vi "Stop Core.vi"(10 "final error code":i32, 11 "Valve in":refnum<class "Valve.lvclass">) -> (3 "Valve out":refnum<class "Valve.lvclass">)   [LabVIEW 2015, in "cRIO-Carbondioxide.lvlib" / "CO2-Actor.lvlib" / "Valve.lvclass"]
doc: "(<B>Filename</B>: Actor Framework.lvlib:Actor.lvclass:Stop Core.vi)\n\nDefines what the actor does before it stops. Use the <B>final error code</B> input to determine whether the actor shut down in response to an error.\n\nBy default, this method does nothing. A descendant class may override it to define behavior, such as shutting down any processes the actor initiated in its override of the Actor Core method."
uses:
  Valve.lvclass
  Valve.lvclass/Valve.ctl
  Interlocks/Interlock Bool/Interlock Bool.lvclass
  CO2 Actor/CO2 Actor.lvclass/CO2 Actor.ctl
  Interlocks/Interlock Chain/Interlock Chain.lvclass/Interlock Chain.ctl
  Interlocks/Interlock/Interlock.lvclass/Interlock.ctl
  Interlocks/Interlock Bool/Interlock Bool.lvclass/Interlock Bool.ctl
  Interlocks/Interlock/Interlock.lvclass
  Interlocks/Interlock Chain/Interlock Chain.lvclass
  CO2 Actor/CO2 Actor.lvclass
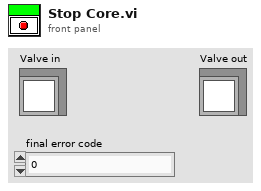
[diagram p1: front panel]
types:
  T1 = typedef "Action.ctl" = enum16{"Open", "Close", "None"}
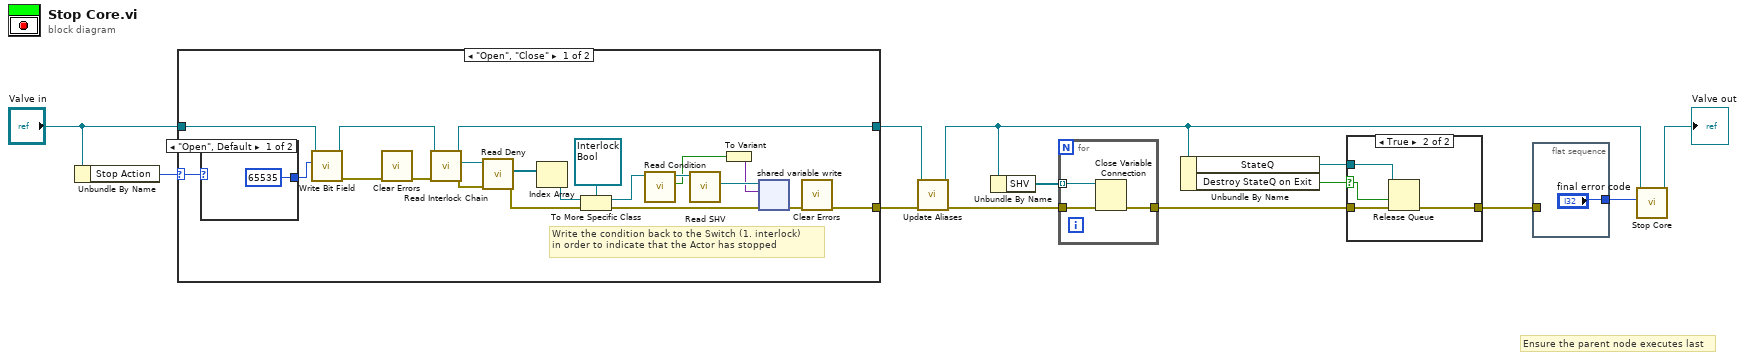
[diagram p0: block diagram]
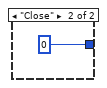
[diagram p3: hidden frame]
diagram:
  # "Ensure the parent node executes last"
  n1 = Unbundle By Name("Valve in") -> ("Stop Action"=w10:T1)
  n2 = case shown="\"Open\", \"Close\"" w10 {
    selector: w10 -> [w23 _]
    tunnel: [w32 _] -> w8
    tunnel: [w17 w37] -> w6
    tunnel: "Valve in" -> [w18 w37]
    frame "Open", "Close" {
      # "Write the condition back to the Switch (1. interlock)\nin order to indicate that the Actor has stopped"
      n3 = case shown="\"Open\", Default" w23 {
        tunnel: [u16 65535 ("Bit Field") u16 0 ("Bit Field")] -> w16
        frame "Open", Default {
        }
        frame "Close" {
        }
      }
      n4 = call "Write Bit Field.vi"("Bit Field"=w16, "Valve in"=w18) -> ("error out"=w14:errorcluster, "Valve out"=w15:refnum<class "Valve.lvclass">)  [unwired: 7 in, 1 out]
      n5 = call <vilib>:"Clear Errors.vi"("error in (no error)"=w14) -> ("error out"=w30:errorcluster)  [unwired: 5 in, 1 out]
      n6 = call "Read Interlock Chain.vi"("error in (no error)"=w30, "CO2 Actor in"=w15) -> ("error out"=w21:errorcluster, "Interlock Chain"=w22:refnum<class "Interlock Chain.lvclass">, "CO2 Actor out"=w17:refnum<class "Valve.lvclass">)  [unwired: 7 in]
      n7 = call "Read Deny.vi"("error in (no error)"=w21, "Interlock Chain in"=w22) -> ("error out"=w20:errorcluster, "Deny"=w19:refnum<class "Interlock.lvclass">[])  [unwired: 7 in, 1 out]
      n8 = Index Array(array=w19) -> (element=w28:refnum<class "Interlock.lvclass">)  [unwired: 1 in]
      n9 = To More Specific Class(target class=refnum<class "Interlock Bool.lvclass"> refnum ("Interlock Bool in"), reference=w28, error in=w20) -> (specific class reference=w25:refnum<class "Interlock Bool.lvclass">, error out=w26:errorcluster)
      n10 = call "Read Condition.vi"("Interlock Bool in"=w25) -> ("Interlock Condition"=w24:bool, "Interlock Bool out"=w29:refnum<class "Interlock Bool.lvclass">)  [unwired: 9 in]
      n11 = call "Read SHV.vi"("Interlock in"=w29) -> ("SHV"=w34:refnum<k21>)  [unwired: 8 in, 2 out]
      n12 = To Variant(anything=w24) -> (Variant=w31:variant)
      n13 = shared-variable-write(w34, w26, w31) -> (w33:errorcluster)  [unwired: 1 out]
      n14 = call <vilib>:"Clear Errors.vi"("error in (no error)"=w33) -> ("error out"=w32:errorcluster)  [unwired: 5 in, 1 out]
    }
    frame "None" {
    }
  }
  n15 = call "Update Aliases.vi"("error in (no error)"=w8, "Valve in"=w6) -> ("error out"=w7:errorcluster, "Valve out"=w5:refnum<class "Valve.lvclass">)  [unwired: 8 in]
  n16 = Unbundle By Name(w5) -> ("SHV"=w9:refnum<k21>[])
  n17 = for {
    tunnel: [w38] -> w3
    tunnel: w7 -> [w40]
    tunnel: w9 -> [w39] mode=indexing
    n18 = Close Variable Connection(8:w40, 11:w39) -> (0:w38:errorcluster)
  }
  n19 = Unbundle By Name(w5) -> ("StateQ"=w4:refnum<queue>, "Destroy StateQ on Exit"=w1:bool)
  n20 = case shown="True" w1 {
    selector: w1 -> [_ w42]
    tunnel: w4 -> [_ w43]
    tunnel: w3 -> [w41 w45]
    tunnel: [w41 w44] -> w2
    frame False {
    }
    frame True {
      n21 = Release Queue(queue=w43, force destroy? (F)=w42, error in (no error)=w45) -> (error out=w44:errorcluster)  [unwired: 2 out]
    }
  }
  n22 = flat-sequence {
    tunnel: ["final error code"] -> w13
    tunnel: w2 -> [_]
    frame #0 {
    }
  }
  n23 = call-parent "Stop Core.vi"("final error code"=w13, "CO2 Actor in"=w5) -> ("CO2 Actor out"=→"Valve out":refnum<class "Valve.lvclass">)  [unwired: 9 in]
